vi "LV2011 - Continously updating radar plot.vi"() -> ()   [LabVIEW 2011]
doc: "Uses the Radar Plot VI to draw a radar plot in a picture indicator."
panel:
  in  "Axis Label":string[](array[string])=["Bolt 1", "Bolt 2", "Bolt 3", "Bolt 4", "Bolt 5", "Bolt 6"]
  in  "Plot Information":T1(array[cluster])=[{"Plot Name"="Bolt Stresses", "Plot Colour"=16449346, "Fill?"=FALSE}]
  in  "Stop Button":bool
  out "Radar Plot":picture
  # "This vi demonstrates using the Radar Plot.vi to visualise data in real time. The Max value for each axis is in the [square bracket]\n1. Run vi 'as is' to see single plot.\n2. Add elements to 'Plot Informtation' to add more plots.\n3. Add elements to 'Axis Label' to add more axis. They are automatically equally spaced."
  # "Each element added to Plot Information\nwill create a new plot. Fill? refers to whether\nor not to just have a line between points."
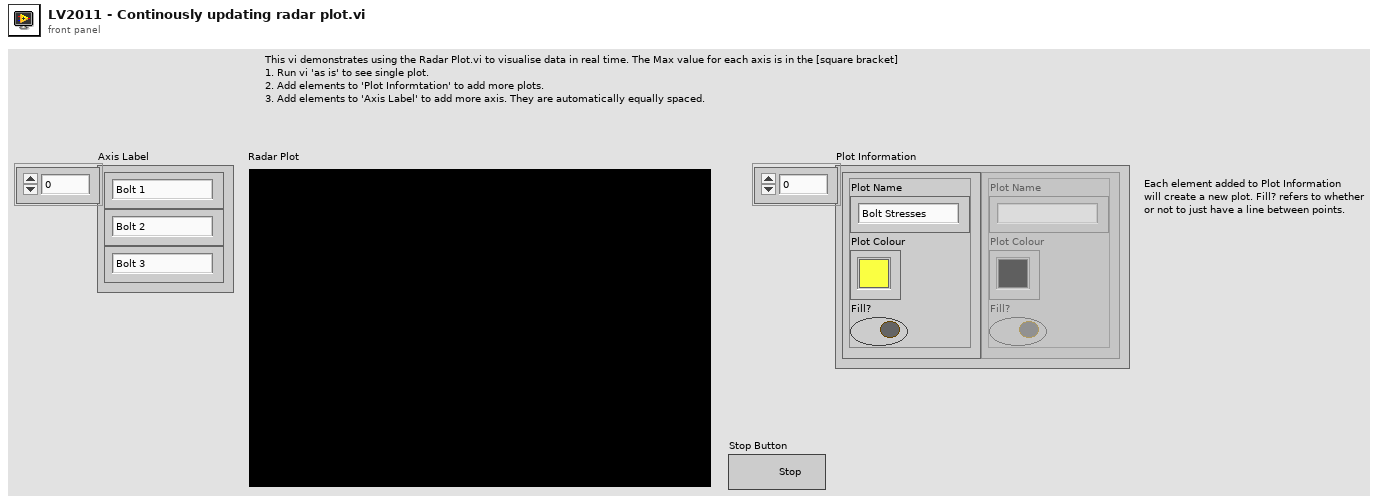
[diagram p1: front panel]
types:
  T1 = cluster{"Plot Name":string, "Plot Colour":u32, "Fill?":bool}[]
  T2 = cluster{"position (none)":enum16{"none", "top", "right", "bottom", "left"}, "text color(white)":u32}
  T3 = cluster{"String":string, "max value":dbl, "min value":dbl}[]
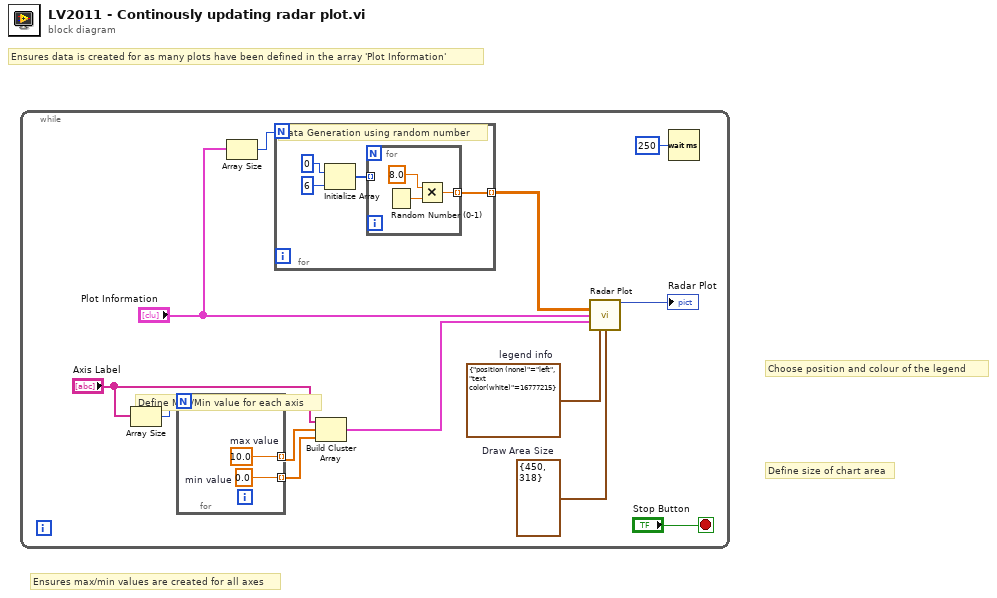
[diagram p0: block diagram]
diagram:
  # "Define size of chart area"
  # "Choose position and colour of the legend"
  # "Ensures max/min values are created for all axes"
  # "Ensures data is created for as many plots have been defined in the array 'Plot Information'"
  n1 = while {
    stop <- "Stop Button" stop-if-true
    w5 = T2 {"position (none)"=enum."left", "text color(white)"=16777215}  # legend info
    w6 = cluster{"Width":u32, "Height":u32} {"Width"=450, "Height"=318}  # Draw Area Size
    n2 = Array Size(array="Axis Label") -> (size(s)=w1:i32)
    n3 = for {
      N: w1 -> [_]
      tunnel: [w21] -> w12 mode=indexing
      tunnel: [w22] -> w11 mode=indexing
      w21 = 10.0  # max value
      w22 = 0.0  # min value
      # "Define Max/Min value for each axis"
    }
    n4 = Array Size(array="Plot Information") -> (size(s)=w3:i32)
    n5 = for {
      N: w3 -> [_]
      tunnel: [w17] -> w9 mode=indexing
      # "Data Generation using random number"
      n6 = Initialize Array(0, 6 ("dimension size")) -> (w14:i32[])
      n7 = for {
        tunnel: [w18] -> w17 mode=indexing
        tunnel: w14 -> [_] mode=indexing
        n8 = Random Number (0-1)() -> (number: 0 to 1=w19:dbl)
        n9 = Multiply(x=8.0, y=w19) -> (x*y=w18:dbl)
      }
    }
    n10 = Build Cluster Array("Axis Label", w12, w11) -> (w10:T3)
    n11 = call <vilib>:"Radar Plot.vi"("data"=w9, "plot info"="Plot Information", "axis info"=w10, "legend info"=w5, "dimension (w,h)"=w6) -> ("new picture"=→"Radar Plot":picture)  [unwired: 10 in]
    n12 = Wait (ms)(milliseconds to wait=u32 250) -> ()  [unwired: 1 out]
  }
